vi "SensorSettings.vi"(2 "Connection In":refnum<k7>) -> (0 "OK Button 2":bool)   [LabVIEW 2025]
uses:
  <vilib>/Utility/config.llb/NI_LVConfig.lvlib
  <vilib>/Utility/config.llb/Read Key (String).vi
  <vilib>/Utility/config.llb/Write Key (String).vi
panel:
  in  "Cancel Button":bool
  in  "OK Button":bool
  in  "Sensor":u16(ring) items=["temp.dg1.1"=3, "temp.dg1.2"=4, "temp.dg1.3"=5, "temp.dg1.4"=6]
  in  "NodeId":string
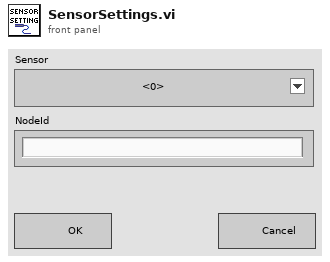
[diagram p1: front panel]
types:
  T1 = typedef "NI_LVConfig.lvlib/Config Data RefNum.ctl" = refnum<k1>
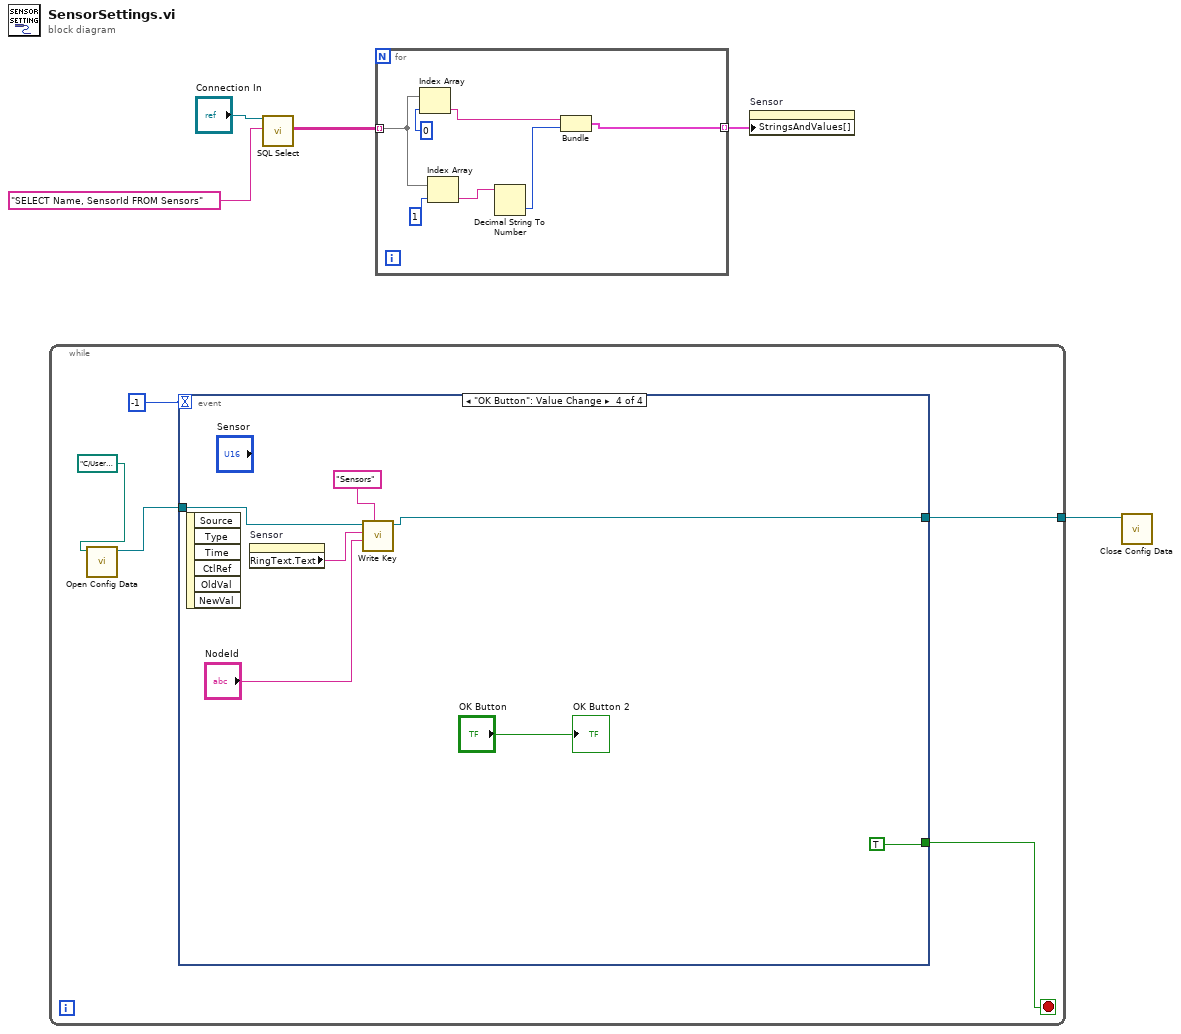
[diagram p0: block diagram]
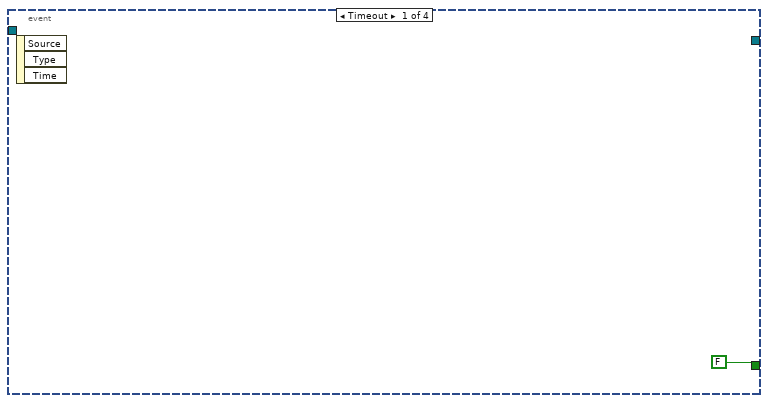
[diagram p2: hidden frame]
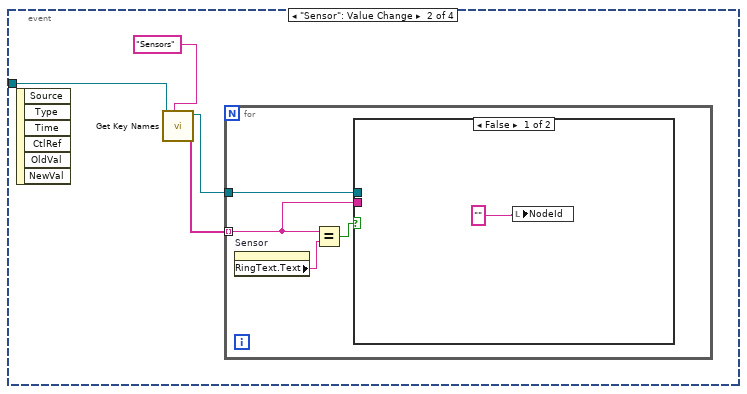
[diagram p3: hidden frame]
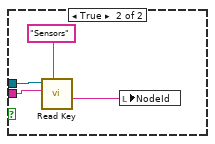
[diagram p4: hidden frame]
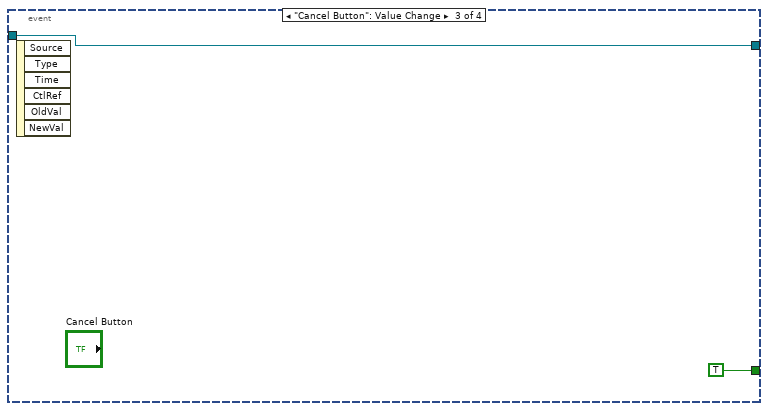
[diagram p5: hidden frame]
diagram:
  n1 = while {
    tunnel: [w6] -> w1
    stop <- w9 stop-if-true
    n2 = call <vilib>:"Open Config Data.vi"("configuration file path"=path "C:/Users/magne/OneDrive/Dokumenter/Skole/IIA2017-1 26V Industrial Information Technology/Assignments/SCADA Assignment/02 Files/Task 3/settings.ini") -> ("refnum"=w8:T1)  [unwired: 8 in, 2 out]
    n3 = event shown="[3] \"OK Button\": Value Change" {
      selector: _ -> [_ _ _ _]
      dyn-events: _ -> [_ _ _ _]
      timeout: -1 -> [_ _ _ _]
      tunnel: [FALSE _ TRUE TRUE] -> w9
      tunnel: w8 -> [_ w12 w25 w33]
      tunnel: [_ _ w25 w29] -> w6
      event Timeout {
        n4 = event-data() -> ()  [unwired: 1 in, 3 out]
      }
      event "Sensor": Value Change {
        n5 = event-data() -> ()  [unwired: 1 in, 6 out]
        n6 = call <vilib>:"Get Key Names.vi"("section"="Sensors", "refnum"=w12) -> ("key names"=w14:string[], "refnum out"=w13:T1)  [unwired: 6 in, 2 out]
        n7 = for {
          tunnel: w14 -> [w16] mode=indexing
          tunnel: w13 -> [w17]
          n8 = property on="Sensor" class="Ring (strict)"() -> ("RingText.Text"=w19:string)  [unwired: 2 in, 2 out]
          n9 = Equal?(x=w16, y=w19) -> (x = y?=w18:bool)
          n10 = case shown="False" w18 {
            tunnel: w17 -> [_ w24]
            tunnel: w16 -> [_ w22]
            frame False {
              n11 = local write "NodeId"("" ("NodeId")) -> ()
            }
            frame True {
              n12 = call-poly <vilib>:"Read Key.vi"("section"="Sensors", "key"=w22, "refnum"=w24) -> ("value"=w21:string)  [unwired: 5 in, 3 out]
              n13 = local write "NodeId"(w21) -> ()
            }
          }
        }
      }
      event "Cancel Button": Value Change {
        n14 = event-data() -> ()  [unwired: 1 in, 6 out]
      }
      event "OK Button": Value Change {
        n15 = event-data() -> ()  [unwired: 1 in, 6 out]
        n16 = property on="Sensor" class="Ring (strict)"() -> ("RingText.Text"=w31:string)  [unwired: 2 in, 2 out]
        n17 = call-poly <vilib>:"Write Key.vi"("section"="Sensors", "value"="NodeId", "key"=w31, "refnum"=w33) -> ("refnum out"=w29:T1)  [unwired: 5 in, 2 out]
        "OK Button 2" <- "OK Button"
      }
    }
  }
  n18 = call <vilib>:"SQL Select.vi"("Connection In"="Connection In", "SQL Query"="SELECT Name, SensorId FROM Sensors") -> ("Data"=w3:string[][])  [unwired: 15 in, 2 out]
  n19 = for {
    tunnel: w3 -> [w40] mode=indexing
    tunnel: [w34] -> w2 mode=indexing
    n20 = Index Array "Index Array"(array=w40, index=0) -> (element=w37:string)
    n21 = Index Array "Index Array"(array=w40, index=1) -> (element=w36:string)
    n22 = Decimal String To Number(string=w36) -> (number=w35:i32)  [unwired: 2 in, 1 out]
    n23 = Bundle("String"=w37, w35) -> (w34:cluster{"String":string, i32})  [unwired: 1 in]
  }
  n24 = property on="Sensor" class="Ring (strict)"("StringsAndValues[]"=w2) -> ()  [unwired: 2 in, 2 out]
  n25 = call <vilib>:"Close Config Data.vi"("refnum"=w1) -> ()  [unwired: 9 in, 2 out]
